vi "Get Subtype Description.vi"(8 "error in (no error)":errorcluster, 11 "Image Assertion in":refnum<class "Image Assertion.lvclass">) -> (0 "error out":errorcluster, 2 "Subtype Description":string, 3 "Image Assertion out":refnum<class "Image Assertion.lvclass">)   [LabVIEW 2020, in "MacroAssert.lvlib" / "Image Assertion.lvclass"]
doc: "Gets the subtype description for <B>Step in</B>, which describes what the step's subtype does specifically."
uses:
  Image Assertion.lvclass
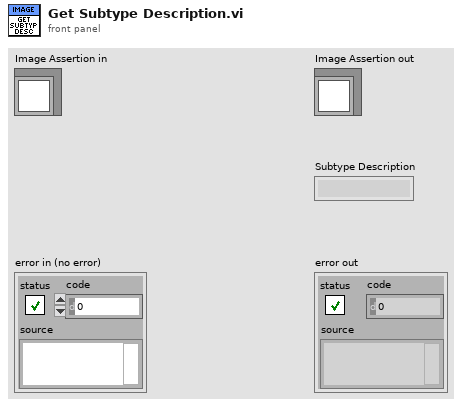
[diagram p1: front panel]
types:
  T1 = typedef "MacroAssert.lvlib/Image Assertion.lvclass/Image Assertion Type.ctl" = enum16{"Control Image", "VI Image", "Window Image"}
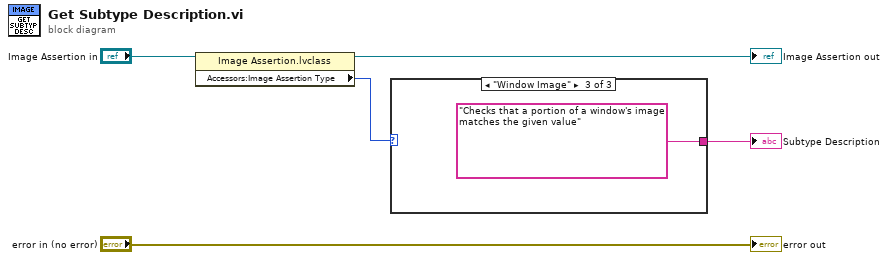
[diagram p0: block diagram]
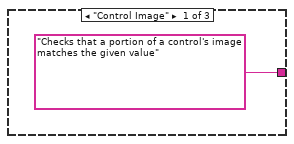
[diagram p2: hidden frame]
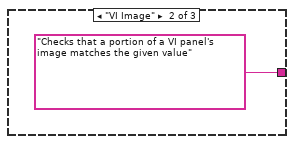
[diagram p3: hidden frame]
diagram:
  n1 = property class="Image Assertion.lvclass"(reference="Image Assertion in") -> (reference out=→"Image Assertion out":refnum<class "Image Assertion.lvclass">, "Accessors:Image Assertion Type"=w5:T1)  [unwired: 1 in, 1 out]
  n2 = case shown="\"Window Image\"" w5 {
    tunnel: ["Checks that a portion of a control's image matches the given value" "Checks that a portion of a VI panel's image matches the given value" "Checks that a portion of a window's image matches the given value"] -> w1
    frame "Control Image" {
    }
    frame "VI Image" {
    }
    frame "Window Image" {
    }
  }
  "Subtype Description" <- w1
  "error out" <- "error in (no error)"
